vi "GetConstantValue.vi"(6 "error in":errorcluster, 9 "Constant in":refnum<class "Constant.lvclass">) -> (0 "error out":errorcluster, 3 "Constant out":refnum<class "Constant.lvclass">, 4 "value":string)   [LabVIEW 2014, in "Raspberry Pi Compatible Compiler for LabVIEW.lvlib" / "Constant.lvclass"]
uses:
  Constant.lvclass
  Python/Parsing/Python Functions.lvlib
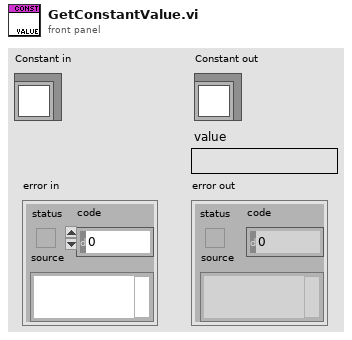
[diagram p1: front panel]
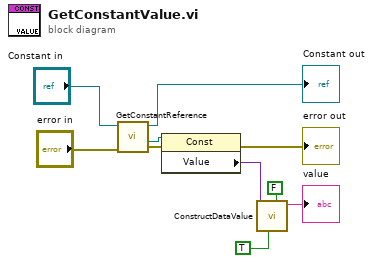
[diagram p0: block diagram]
diagram:
  n1 = call "GetConstantReference.vi"("error in"="error in", "Constant in"="Constant in") -> ("error out"=w7:errorcluster, "reference out"=w6:refnum<vi>, "Constant out"=→"Constant out":refnum<class "Constant.lvclass">)  [unwired: 5 in]
  n2 = property class="Const"(reference=w6, error in=w7) -> (error out=→"error out":errorcluster, "Value"=w10:variant)  [unwired: 1 out]
  n3 = call "ConstructDataValue.vi"("label"=FALSE, "value"=TRUE, "Value"=w10) -> ("value"=→"value":string)  [unwired: 5 in, 1 out]
